vi "dialog_wait_demo.vi"() -> ()   [LabVIEW 2020, in "varilib.lvlib"]
doc: "Simple demonstration of assynchronously called dialogs."
uses:
  varilib.lvlib
  dialog_wait_type.ctl
panel:
  in  "dialog type (single line)":T1
  in  "title string":string="Please wait ..."
  in  "message string":string="Please wait, generating report ..."
  in  "milliseconds to wait":u32=1000
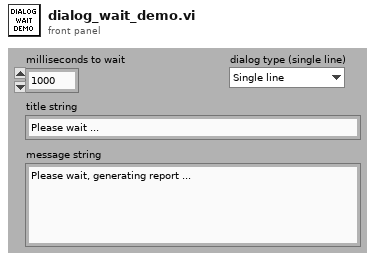
[diagram p1: front panel]
types:
  T1 = typedef "varilib.lvlib/dialog_wait_type.ctl" = enum16{"Single line", "Multi line"}
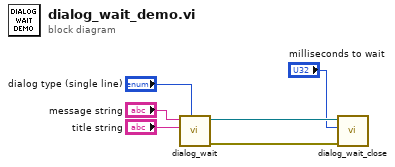
[diagram p0: block diagram]
diagram:
  n1 = call "dialog_wait.vi"("dialog type (single line)"="dialog type (single line)", "title string"="title string", "message string"="message string") -> ("error out"=w6:errorcluster, "reference out"=w3:refnum<vi>)  [unwired: 7 in]
  n2 = call "dialog_wait_close.vi"("error in"=w6, "milliseconds to wait"="milliseconds to wait", "async vi ref"=w3) -> ()  [unwired: 1 in]
